vi "Intake Immediate.vi"(6 "Wait for Manipulator":bool, 7 "Description":string, 8 "Command Info In":T2, 11 "intake modes":T1) -> (0 "Command Info Out":T2)   [LabVIEW 2020]
doc: "This template is useful for immediate subsystem actions that do not need deadband filtering\n\nBe sure to right-click and select New from Template and save with a new command name."
uses:
  <vilib>/Rock Robotics/WPI/Framework/Command Status Info.ctl
  <vilib>/Rock Robotics/WPI/Framework/Completion Status.ctl
  <vilib>/Rock Robotics/WPI/Framework/Completion Notifier.ctl
  Implementation/Typedef/intake typedef.ctl
  Implementation/intake sub Setpoints.ctl
  Implementation/intake sub Operations.ctl
  Framework/Robot Global Data.vi
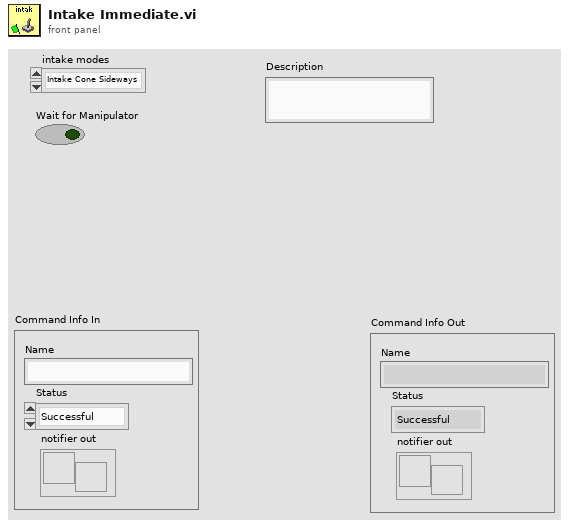
[diagram p1: front panel]
types:
  T1 = typedef "intake typedef.ctl" = enum16{"Intake Cone Sideways", "Intake Cone Upright", "Intake Cube", "Outtake/Score", "Shoot"}
  T2 = typedef "Command Status Info.ctl" = cluster{"Name":string, "Status":T3, "notifier out":T4}
  T3 = typedef "Completion Status.ctl" = enum16{"Successful", "Aborted", "Incomplete"}
  T4 = typedef "Completion Notifier.ctl" = refnum<notifier>
  T5 = typedef "intake sub Setpoints.ctl" = cluster{"Operation":T6, "intake modes":T1}
  T6 = typedef "intake sub Operations.ctl" = enum16{"Reserve", "Read Current", "Immediate"}
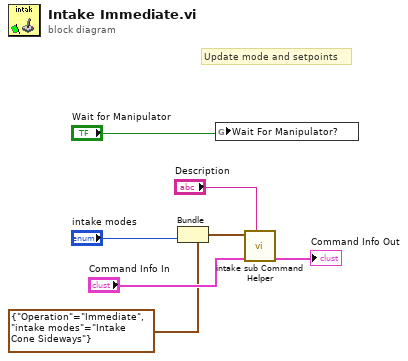
[diagram p0: block diagram]
diagram:
  # "Update mode and setpoints"
  n1 = Bundle(cluster=T5 {"Operation"=enum."Immediate", "intake modes"=enum."Intake Cone Sideways"} ("SubSystem Data"), "intake modes"="intake modes") -> (w4:T5)  [unwired: 1 in]
  n2 = global write "Robot Global Data.vi" "Wait For Manipulator?"("Wait for Manipulator") -> ()
  n3 = call "intake sub Command Helper.vi"("Description"="Description", "Command Info In"="Command Info In", "SubSystem Data"=w4) -> ("Command Info Out"=→"Command Info Out":T2)  [unwired: 6 in, 2 out]
